vi "cdex_Wait Until Next s.vi"(0 "millisecond multiple":dbl=100.0) -> ()   [LabVIEW 2009]
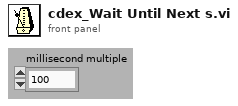
[diagram p1: front panel]
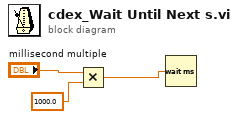
[diagram p0: block diagram]
diagram:
  n1 = Multiply(x="millisecond multiple", y=1000.0) -> (x*y=w2:dbl)
  n2 = Wait (ms)(milliseconds to wait=w2) -> ()  [unwired: 1 out]
